vi "CAEN_HV_subvi_read_withouttimeloop2012.vi"(0 "handle HV1":i32, 1 "handle HV2":i32) -> (2 "Time&Voltage HV1":string[](array[string]), 3 "handle HV1 out":i32, 4 "handle HV2 out":i32, 5 "Time&Voltage HV2":string[](array[string]))   [LabVIEW 2012]
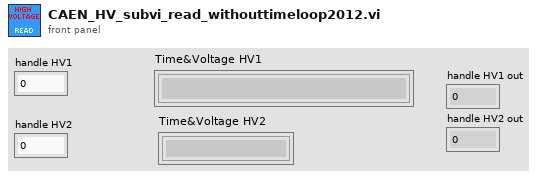
[diagram p1: front panel]
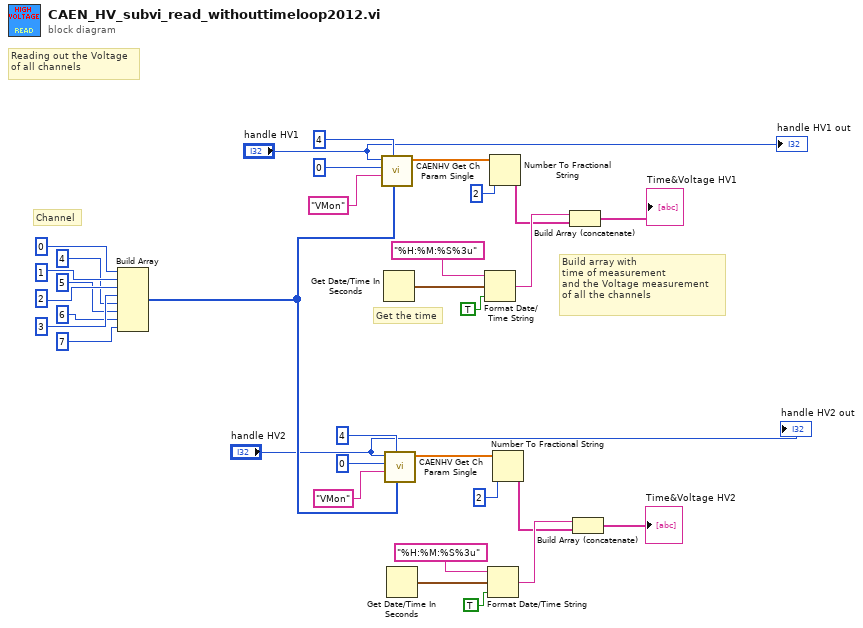
[diagram p0: block diagram]
diagram:
  # "Build array with \ntime of measurement \nand the Voltage measurement \nof all the channels"
  # "Get the time"
  # "Channel"
  # "Reading out the Voltage\nof all channels"
  n1 = Build Array(0, 1, 2, 3, 4, 5, 6, 7) -> (w29:i32[])
  n2 = call "CAENHV Get Ch Param Single.vi"("ChList"=w29, "ChNum (1)"=u16 4, "ParName"="VMon", "slot"=u16 0, "handle"="handle HV1") -> ("ParValList"=w25:sgl[])  [unwired: 5 in, 1 out]
  n3 = Get Date/Time In Seconds() -> (seconds since 1Jan1904=w28:timestamp)
  n4 = call "CAENHV Get Ch Param Single.vi"("ChList"=w29, "ChNum (1)"=u16 4, "ParName"="VMon", "slot"=u16 0, "handle"="handle HV2") -> ("ParValList"=w15:sgl[])  [unwired: 5 in, 1 out]
  n5 = Get Date/Time In Seconds() -> (seconds since 1Jan1904=w18:timestamp)
  n6 = Format Date/Time String(time format string (%c)="%H:%M:%S%3u", seconds (now)=w28, UTC format=TRUE ("want seconds? (F)")) -> (date/time string=w27:string)
  n7 = Format Date/Time String(time format string (%c)="%H:%M:%S%3u", seconds (now)=w18, UTC format=TRUE ("want seconds? (F)")) -> (date/time string=w17:string)
  n8 = Number To Fractional String(number=w25, precision (6)=i16 2) -> (F-format string=w24:string[])  [unwired: 2 in]
  n9 = Number To Fractional String(number=w15, precision (6)=i16 2) -> (F-format string=w14:string[])  [unwired: 2 in]
  n10 = Build Array (concatenate)(w27, w24) -> (→"Time&Voltage HV1":string[])
  n11 = Build Array (concatenate)(w17, w14) -> (→"Time&Voltage HV2":string[])
  "handle HV1 out" <- "handle HV1"
  "handle HV2 out" <- "handle HV2"
